vi "P01_Filtro promediador.vi"() -> ()   [LabVIEW 2026]
panel:
  out "Numeric":dbl
  out "Array":dbl[](array[numeric])
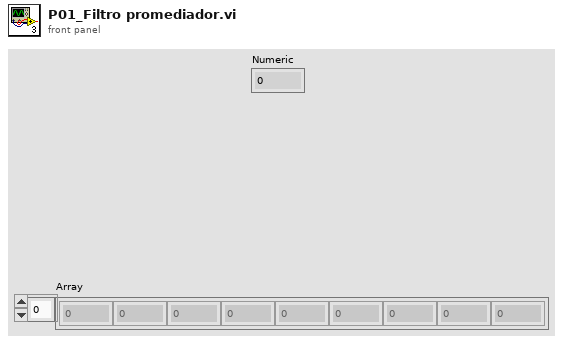
[diagram p1: front panel]
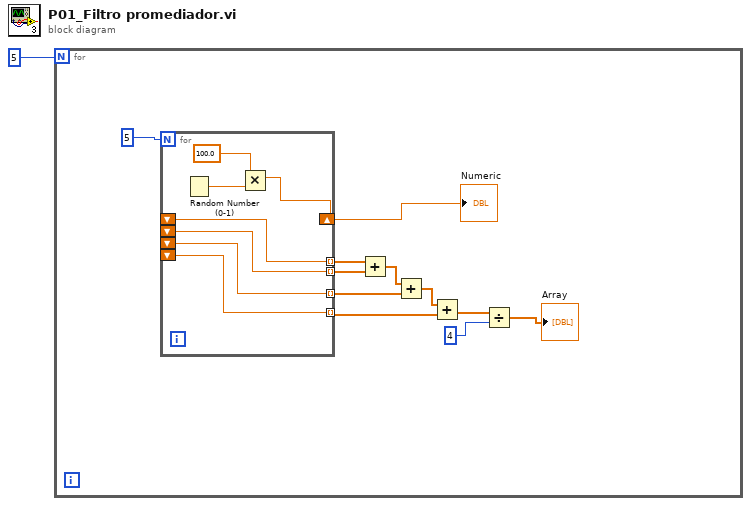
[diagram p0: block diagram]
diagram:
  n1 = for {
    N: 5 -> [_]
    n2 = for {
      N: 5 -> [_]
      shift-right: [w17] -> w11
      shift-left: _ -> [w16]
      shift-left: _ -> [w15]
      shift-left: _ -> [w14]
      shift-left: _ -> [w13]
      tunnel: [w16] -> w10 mode=indexing
      tunnel: [w15] -> w9 mode=indexing
      tunnel: [w14] -> w7 mode=indexing
      tunnel: [w13] -> w5 mode=indexing
      n3 = Random Number (0-1)() -> (number: 0 to 1=w19:dbl)
      n4 = Multiply(x=100.0, y=w19) -> (x*y=w17:dbl)
    }
    "Numeric" <- w11
    n5 = Add(x=w10, y=w9) -> (x+y=w8:dbl[])
    n6 = Add(x=w8, y=w7) -> (x+y=w6:dbl[])
    n7 = Add(x=w6, y=w5) -> (x+y=w4:dbl[])
    n8 = Divide(x=w4, y=4) -> (x/y=→"Array":dbl[])
  }
